vi "PV ActiveLine - DisplayControlBargraph.vi"(7 "W/R":bool, 8 "Fehler (Eingang)":errorcluster, 9 "Bargraph Mode":i8 min=0 max=10, 11 "Referenz in":refnum<visa-resource-name>) -> (0 "Cluster (Ausgang)":errorcluster, 1 "Bargraph Mode Out":i8, 3 "Referenz out":refnum<visa-resource-name>)   [LabVIEW 2013, in "PV ActiveLine.lvlib"]
doc: "DCB - Display Control Bar Graph\n\nTransmit: DCB [,a]\n\nBar graph display,\na =\n0 –> Off (default)\n1 –> Bar graph covering full scale range\n2 –> Bar graph covering full scale range, high-level presentation\n3 –> Bar graph covering full scale range and setpoint threshold\n4 –> Bar graph covering a decade according to current measurement value\n5 –> Bar graph covering a decade according to current measurement value, high-level presentation\n6 –> Bar graph covering a decade according to current measurement value and setpoint threshold\n7 –> p = f(t), autoscaled, 0.2 seconds / pixel. For each measurement every 200 ms a measurement value is saved in tabular form and the last 100 measurement values (=100 pixel) are shown autoscaled. The represented data string corresponds to a logging duration of 20 seconds.\n8 –> p = f(t), autoscaled, 1 second / pixel. For each measurement every second a measurement value is saved in tabular form and the last 100 measurement values (=100 pixel) are shown autoscaled. The represented data string corresponds to a logging duration of 100 seconds.\n9 –> p = f(t), autoscaled, 6 seconds / pixel. For each measurement every 6 seconds a\nmeasurement value is saved in tabular form and the last 100 measurement values (=100 pixel) are shown autoscaled. The represented data string corresponds to a logging duration of 10 minutes.\n10 –> p = f(t), autoscaled, 1 minute / pixel. For each measurement every minute a measurement value is saved in tabular form and the last 100 measurement values (=100 pixel) are shown autoscaled. The represented data string corresponds to a logging duration of 100 minutes."
uses:
  <instrlib>/PV ActiveLine/PV ActiveLine.lvlib
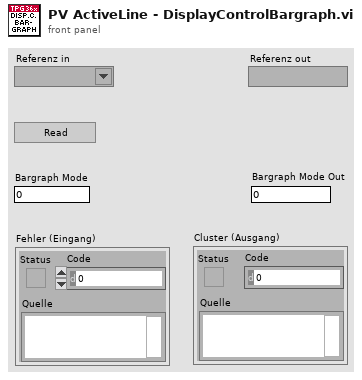
[diagram p1: front panel]
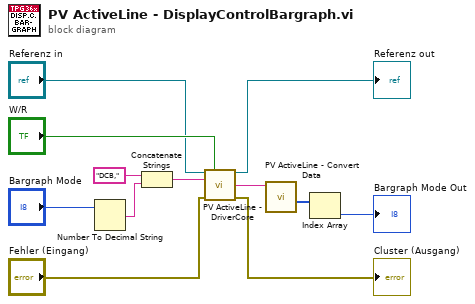
[diagram p0: block diagram]
diagram:
  n1 = Number To Decimal String(number="Bargraph Mode") -> (decimal integer string=w9:string)  [unwired: 1 in]
  n2 = Concatenate Strings("DCB,", w9) -> (w10:string)
  n3 = call <instrlib>:"PV ActiveLine - DriverCore.vi"("Referenz in"="Referenz in", "Write/Read"="W/R", "Command"=w10, "Fehler (Eingang)"="Fehler (Eingang)") -> ("Referenz out"=→"Referenz out":refnum<visa-resource-name>, "String Out"=w3:string, "Cluster (Ausgang)"=→"Cluster (Ausgang)":errorcluster)  [unwired: 9 in]
  n4 = call <instrlib>:"PV ActiveLine - Convert Data.vi"("String in"=w3) -> ("Integer Out"=w2:i32[])  [unwired: 7 in, 3 out]
  n5 = Index Array(array=w2) -> (element=→"Bargraph Mode Out":i32)  [unwired: 1 in]
